vi "configure operation.vi"(7 "EthernetIP configuration":refnum<class "EthernetIP configuration.lvclass">, 8 "error in":errorcluster, 10 "line item in":T2, 11 "engine configuration in":refnum<class "engine configuration.lvclass">) -> (0 "error out":errorcluster, 1 "success":bool, 2 "line item out":T2, 5 "changed":bool)   [LabVIEW 2013, in "EthernetIP editor node.lvclass"]
uses:
  EthernetIP editor node.lvclass
  table line.ctl
  channel/EthernetIP Channel.lvclass
  <vilib>/NI/Module Execution Interface/Engine Configuration/engine configuration.lvclass
  configuration/EthernetIP configuration.lvclass
  <vilib>/NI/Tag Bus/tag/Data Type.ctl
  configuration/EthernetIP configuration.lvclass/EthernetIP configuration.ctl
  <vilib>/NI/Configuration Framework/serializable configuration/NISE_CEF_serializable configuration.lvclass/NISE_CEF_serializable configuration.ctl
  <vilib>/NI/Tag Bus/tag/tag descriptor.lvclass/tag descriptor.ctl
  channel/EthernetIP Channel.lvclass/EthernetIP Channel.ctl
  <vilib>/NI/Tag Bus Module Framework/channel/TBM channel.lvclass/TBM channel.ctl
  configuration/Read assemblies.vi
  <vilib>/NI/Configuration Framework/serializable configuration/Read UID.vi
  <vilib>/NI/Tag Bus Module Framework/channel/Read channel classification.vi
  <vilib>/NI/Tag Bus/tag/read tag name.vi
  <vilib>/NI/Tag Bus/tag/read data type.vi
  channel/Read byte index.vi
  channel/Read Instance ID.vi
  <vilib>/NI/Tag Bus/tag/write tag name.vi
  channel/Write Instance ID.vi
  <vilib>/NI/Tag Bus Module Framework/channel/Write channel classification.vi
  <vilib>/NI/Tag Bus/tag/write data type.vi
  channel/Write byte index.vi
  <vilib>/Utility/LVClass/Get LV Class Name.vi
  <vilib>/NI/Configuration Framework/error generator.vi
  <vilib>/NI/Tag Bus/tag/tag descriptor.lvclass
panel:
  out "Instance data type":T1=enum."Boolean"
  in  "refresh tags":bool
  in  "Tag":i32(listbox)
  in  "Instance":i32(listbox)
  out "problem":string
  in  "Element Index":i32
  in  "Channel Name":string
  in  "cancel":bool
  in  "ok":bool
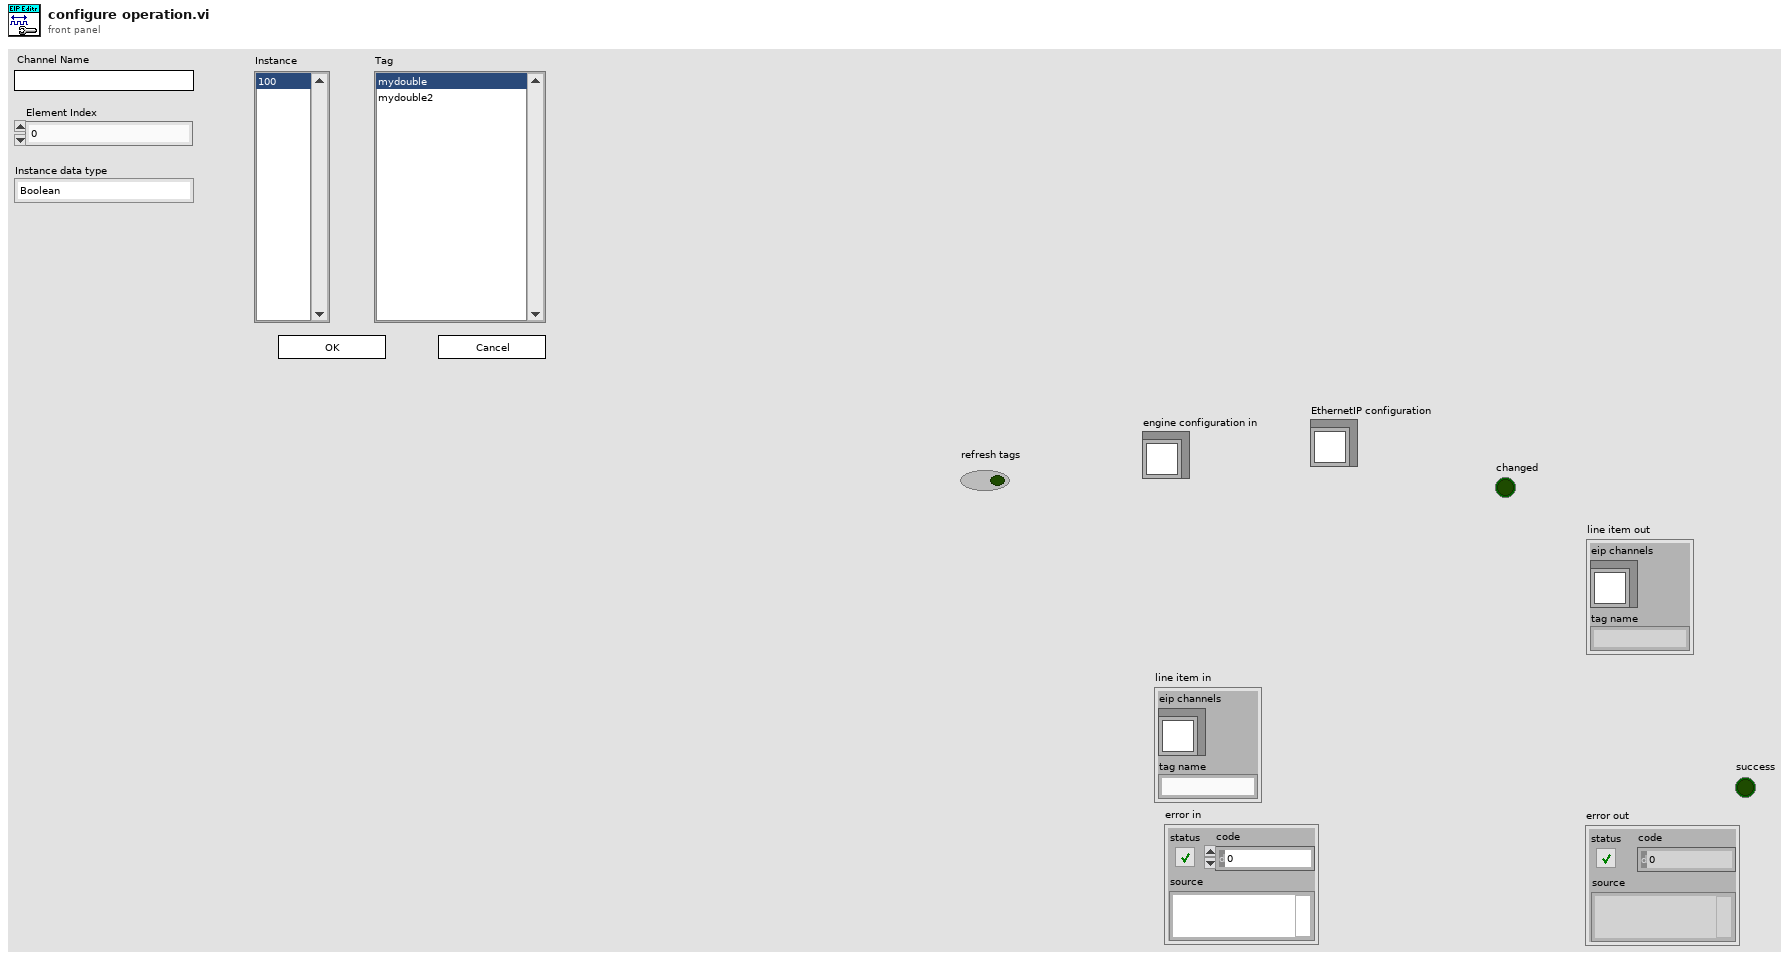
[diagram p1: front panel]
types:
  T1 = typedef "tag bus.lvlib/tag descriptor.lvclass/Data Type.ctl" = enum16{"Double", "Single", "I64", "I32", "I16", "I8", "U64", "U32", "U16", "U8", "Boolean", "String", "Array of Double", "Array of Single", "Array of I64", "Array of I32", "Array of I16", "Array of I8", "Array of U64", "Array of U32", "Array of U16", "Array of U8", "Array of Boolean", "Array of String"}
  T2 = typedef "EthernetIP editor node.lvclass/table line.ctl" = cluster{"eip channels":refnum<class "EthernetIP Channel.lvclass">, "tag name":string}
  T3 = enum32{"Invalid", "Standard", "Closed", "Hidden", "Minimized", "Maximized"}
  T4 = enum32{"Invalid", "Default", "Floating", "Floating/Auto-Hide", "Modal"}
  T5 = enum8{"Enabled", "Disabled", "Disabled and Grayed Out"}
  T6 = typedef "EthernetIP configuration.lvclass/assembly definition.ctl" = cluster{"name":string, "Instance ID":u32, "Type":T7, "Size (elements)":u32, "big endian?":bool, "data type":T1}
  T7 = typedef "EthernetIP configuration.lvclass/assembly type.ctl" = enum32{"Producing", "Consuming"}
  T8 = enum32{"invalid app kind", "Development System", "Run Time System", "Student Edition", "Embedded LabVIEW", "Evaluation", "Custom"}
  T9 = typedef "TBM channel.lvclass/channel classification.ctl" = enum16{"input data", "output data", "processing parameter", "processing result"}
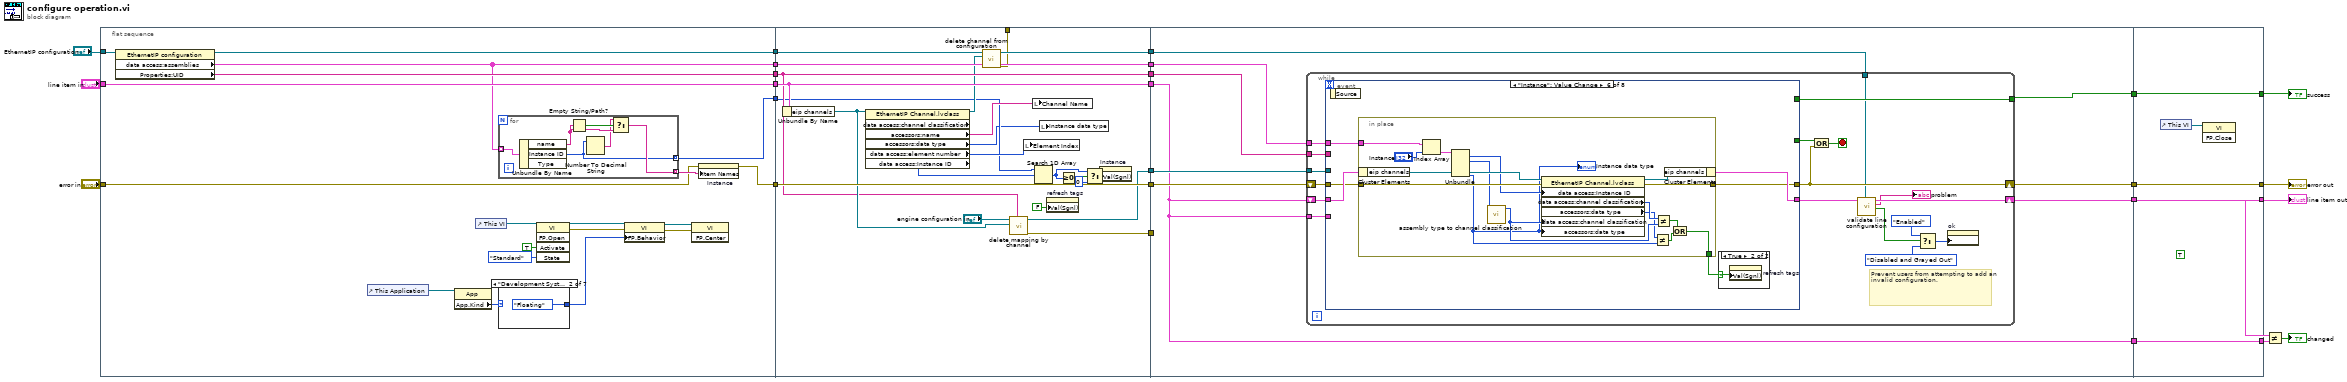
[diagram p0: block diagram]
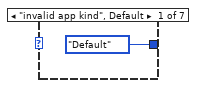
[diagram p2: hidden frame]
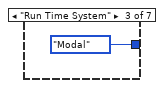
[diagram p3: hidden frame]
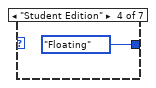
[diagram p4: hidden frame]
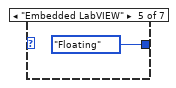
[diagram p5: hidden frame]
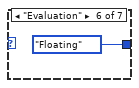
[diagram p6: hidden frame]
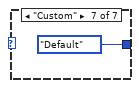
[diagram p7: hidden frame]
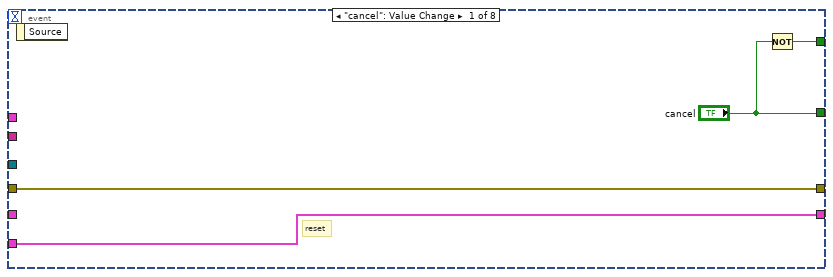
[diagram p8: hidden frame]
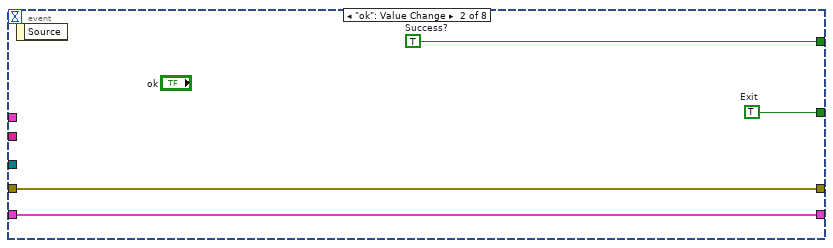
[diagram p9: hidden frame]
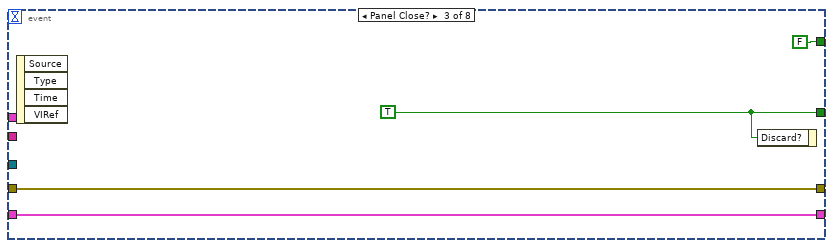
[diagram p10: hidden frame]
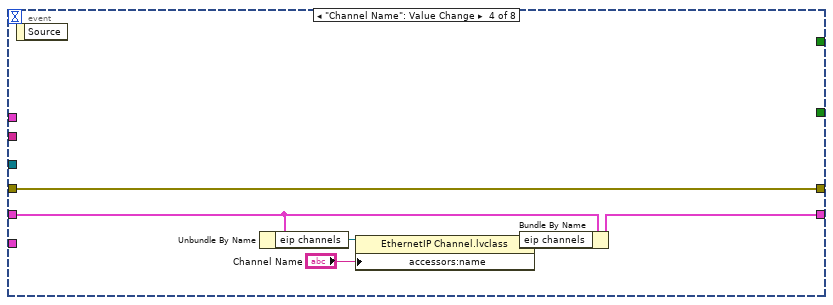
[diagram p11: hidden frame]
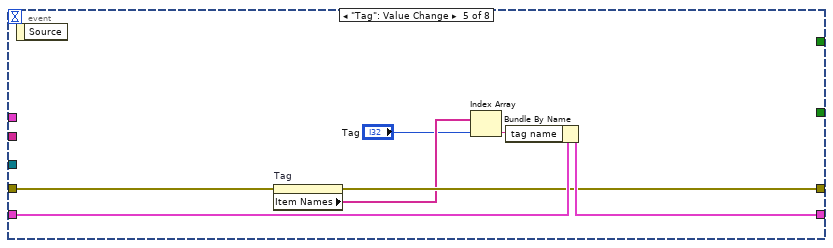
[diagram p12: hidden frame]
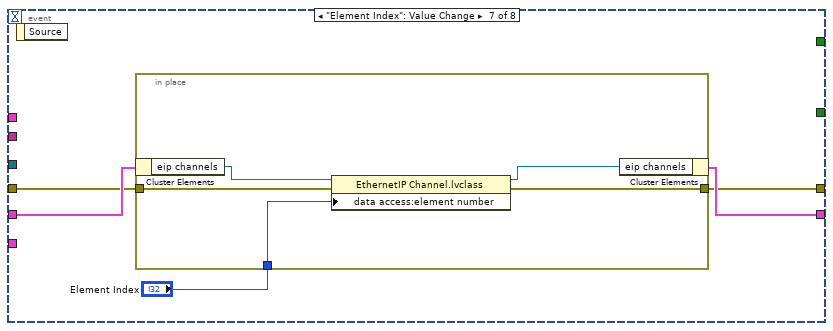
[diagram p14: hidden frame]
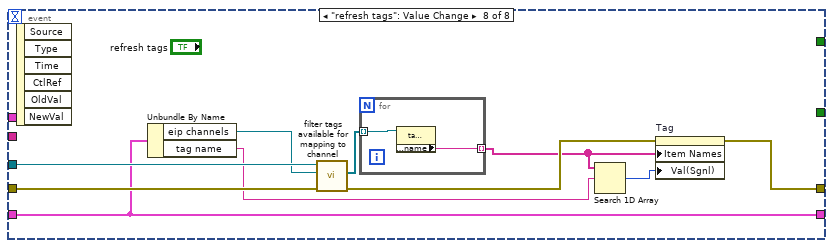
[diagram p15: hidden frame]
diagram:
  n1 = flat-sequence {
    tunnel: "line item in" -> [w44]
    tunnel: "error in" -> [w30]
    tunnel: [w29] -> w14
    tunnel: [w44] -> w12
    tunnel: "EthernetIP configuration" -> [w35]
    tunnel: [w34] -> w6
    tunnel: [w32] -> w4
    tunnel: [w33] -> w3
    tunnel: [w28] -> w1
    tunnel: w14 -> [w79]
    tunnel: [w79] -> w13
    tunnel: w12 -> [w77]
    tunnel: [w77] -> w11
    tunnel: [w75] -> w10
    tunnel: [w74] -> w9
    tunnel: [w68] -> w7
    tunnel: w6 -> [w71]
    tunnel: [w70] -> w5
    tunnel: w4 -> [w70]
    tunnel: w3 -> [w69]
    tunnel: [w69] -> w2
    tunnel: [w66] -> _
    tunnel: w1 -> [w65]
    tunnel: [w87] -> w18
    tunnel: [w86] -> w17
    tunnel: [w85] -> w16
    tunnel: [w80] -> w15
    tunnel: w13 -> [w88]
    tunnel: w11 -> [w80]
    tunnel: w10 -> [_]
    tunnel: w9 -> [w84]
    tunnel: w7 -> [w83]
    tunnel: w5 -> [w82]
    tunnel: w2 -> [w81]
    tunnel: [w177] -> w19
    tunnel: [w178] -> w22
    tunnel: [w179] -> w23
    tunnel: [w180] -> w24
    tunnel: w18 -> [w180]
    tunnel: w17 -> [w179]
    tunnel: w16 -> [w178]
    tunnel: w15 -> [w177]
    frame #0 {
      n2 = property class="EthernetIP configuration"(reference=w35) -> (reference out=w34:refnum<class "EthernetIP configuration.lvclass">, "data access:assemblies"=w32:T6[], "Properties:UID"=w33:string)  [unwired: 1 in, 1 out]
      n3 = control-ref of="This Application"() -> (w38:refnum<vi>)
      n4 = property class="App"(reference=w38) -> ("App.Kind"=w37:T8)  [unwired: 1 in, 2 out]
      n5 = control-ref of="This VI"() -> (w39:refnum<vi>)
      n6 = for {
        tunnel: w32 -> [w50] mode=indexing
        tunnel: [w46] -> w31 mode=indexing
        tunnel: [w45] -> w28 mode=indexing
        n7 = Unbundle By Name(w50) -> ("name"=w48:string, "Instance ID"=w45:u32)  [unwired: 1 out]
        n8 = Empty String/Path?(string/path=w48) -> (empty?=w49:bool)
        n9 = Number To Decimal String(number=w45) -> (decimal integer string=w47:string)  [unwired: 1 in]
        n10 = Select(t=w47, s=w49, f=w48) -> (s? t:f=w46:string)
      }
      n11 = case shown="\"Development System\"" w37 {
        tunnel: [T4."Default" ("Front Panel Window:Behavior") T4."Floating" ("Front Panel Window:Behavior") T4."Modal" ("Front Panel Window:Behavior") T4."Floating" ("Front Panel Window:Behavior") T4."Floating" ("Front Panel Window:Behavior") T4."Floating" ("Front Panel Window:Behavior") T4."Default" ("Front Panel Window:Behavior")] -> w36
        frame "invalid app kind", Default {
        }
        frame "Development System" {
        }
        frame "Run Time System" {
        }
        frame "Student Edition" {
        }
        frame "Embedded LabVIEW" {
        }
        frame "Evaluation" {
        }
        frame "Custom" {
        }
      }
      n12 = invoke class="VI" method="FP.Open"(reference=w39, "Activate"=TRUE ("Activate?"), "State"=T3."Standard") -> (reference out=w42:refnum<vi>, error out=w43:errorcluster)  [unwired: 2 in, 3 out]
      n13 = property class="VI"(reference=w42, error in=w43, "FP.Behavior"=w36) -> (reference out=w27:refnum<vi>, error out=w26:errorcluster)
      n14 = invoke class="VI" method="FP.Center"(reference=w27, error in=w26) -> ()  [unwired: 1 in, 3 out]
      n15 = property on="Instance" class="LstBox (strict)"(error in=w30, "Item Names"=w31) -> (error out=w29:errorcluster)  [unwired: 1 in, 1 out]
    }
    frame #1 {
      n16 = Unbundle By Name(w77) -> ("eip channels"=w73:refnum<class "EthernetIP Channel.lvclass">)
      n17 = property class="EthernetIP Channel.lvclass" props=["data access:channel classification", "accessors:name", "accessors:data type", "data access:element number", "data access:Instance ID"](reference=w73) -> (reference out=w67:refnum<class "EthernetIP Channel.lvclass">, "accessors:name"=w78:string, "accessors:data type"=w58:T1, "data access:element number"=w72:i32, "data access:Instance ID"=w60:u32)  [unwired: 1 in, 2 out]
      n18 = call "delete channel from configuration.vi"("TBM channel in"=w67, "EthernetIP configuration in"=w71) -> ("error out"=w66:errorcluster, "EthernetIP configuration out"=w68:refnum<class "EthernetIP configuration.lvclass">)  [unwired: 8 in]
      n19 = call <vilib>:"delete mapping by channel.vi"("owner ID"=w69, "channel"=w73, "engine configuration in"="engine configuration in") -> ("error out"=w75:errorcluster, "engine configuration out"=w74:refnum<class "engine configuration.lvclass">)  [unwired: 7 in]
      n20 = local write "Element Index"(w72) -> ()
      n21 = local write "Channel Name"(w78) -> ()
      n22 = Search 1D Array(1D array=w65, element=w60) -> (index of element=w62:i32)  [unwired: 1 in]
      n23 = local write "Instance data type"(w58) -> ()
      n24 = property on="refresh tags" class="Bool (strict)"("Val(Sgnl)"=FALSE ("Value (Signaling)")) -> ()  [unwired: 2 in, 2 out]
      n25 = Greater Or Equal To 0?(x=w62) -> (x >= 0?=w63:bool)
      n26 = Select(t=w62, s=w63, f=0) -> (s? t:f=w61:i32)
      n27 = property on="Instance" class="LstBox (strict)"("Val(Sgnl)"=w61) -> ()  [unwired: 2 in, 2 out]
    }
    frame #2 {
      n28 = while {
        shift-right: [w97] -> w86
        shift-left: w88 -> [w105]
        tunnel: [w104] -> w87
        shift-right: [w98] -> w85
        shift-left: w80 -> [w101]
        tunnel: w80 -> [w100]
        tunnel: w84 -> [w106]
        tunnel: w83 -> [w92]
        tunnel: w82 -> [w91]
        tunnel: w81 -> [w90]
        stop <- w102 stop-if-true
        # "Prevent users from attempting to add an invalid configuration."
        n29 = event shown="[5] \"Instance\": Value Change" {
          selector: _ -> [_ _ _ _ _ _ _ _]
          dyn-events: _ -> [_ _ _ _ _ _ _ _]
          timeout: _ -> [_ _ _ _ _ _ _ _]
          tunnel: w106 -> [_ _ _ _ _ _ _ w171]
          tunnel: w105 -> [w110 w114 w118 w124 w130 w135 w157 w173]
          tunnel: [w110 w114 w118 w124 w127 w134 w156 w172] -> w97
          tunnel: [w109 w111 FALSE _ _ _ _ _] -> w104
          tunnel: ["cancel" w112 w116 _ _ _ _ _] -> w103
          tunnel: w101 -> [_ w113 w115 w122 w131 w137 w159 w170]
          tunnel: [w107 w113 w115 w123 w129 w136 w158 w170] -> w99
          tunnel: w100 -> [w107 _ _ _ _ _ _ _]
          tunnel: w91 -> [_ _ _ _ _ w132 _ _]
          tunnel: w90 -> [_ _ _ _ _ _ _ _]
          event "cancel": Value Change {
            # "reset"
            n30 = event-data() -> ()  [unwired: 1 in, 1 out]
            n31 = Not(x="cancel") -> (.not. x?=w109:bool)
          }
          event "ok": Value Change {
            w111 = TRUE  # Success?
            w112 = TRUE  # Exit
            n32 = event-data() -> ()  [unwired: 1 in, 1 out]
          }
          event Panel Close? {
            w116 = TRUE ("cancel")
            n33 = event-data() -> ()  [unwired: 1 in, 4 out]
            n34 = event-data("Discard?"=w116) -> ()  [unwired: 1 in, 1 out]
          }
          event "Channel Name": Value Change {
            n35 = event-data() -> ()  [unwired: 1 in, 1 out]
            n36 = Unbundle By Name(w122) -> ("eip channels"=w121:refnum<class "EthernetIP Channel.lvclass">)
            n37 = property class="EthernetIP Channel.lvclass"(reference=w121, "accessors:name"="Channel Name") -> (reference out=w120:refnum<class "EthernetIP Channel.lvclass">)  [unwired: 1 in, 1 out]
            n38 = Bundle By Name(cluster=w122, "eip channels"=w120) -> (w123:T2)
          }
          event "Tag": Value Change {
            n39 = event-data() -> ()  [unwired: 1 in, 1 out]
            n40 = property on="Tag" class="LstBox (strict)"(error in=w130) -> (error out=w127:errorcluster, "Item Names"=w126:string[])  [unwired: 1 in, 1 out]
            n41 = Index Array(array=w126, index="Tag") -> (element=w128:string)
            n42 = Bundle By Name(cluster=w131, "tag name"=w128) -> (w129:T2)
          }
          event "Instance": Value Change {
            n43 = event-data() -> ()  [unwired: 1 in, 1 out]
            n44 = in-place {
              in-place-border: w135 -> [w154]
              in-place-border: [w153] -> w134
              in-place-border: [w140] -> w133
              in-place-border: w132 -> [w147]
              n45 = in-place-cluster #1(w137) -> ("eip channels"=w152:refnum<class "EthernetIP Channel.lvclass">)
              n46 = Index Array(array=w147, index="Instance") -> (element=w146:T6)
              n47 = Unbundle(w146) -> ("Instance ID"=w145:u32, "Type"=w144:T7, "data type"=w139:T1)  [unwired: 3 out]
              "Instance data type" <- w139
              n48 = call "assembly type to channel classification.vi"("Type"=w144) -> ("channel classification"=w149:T9)  [unwired: 10 in]
              n49 = property class="EthernetIP Channel.lvclass"(reference=w152, error in=w154, "data access:Instance ID"=w145, "data access:channel classification"=w149, "accessors:data type"=w139) -> (reference out=w151:refnum<class "EthernetIP Channel.lvclass">, error out=w153:errorcluster, "data access:channel classification"=w150:T9, "accessors:data type"=w143:T1)
              n50 = Not Equal?(x=w143, y=w139) -> (x != y?=w142:bool)
              n51 = Not Equal?(x=w150, y=w149) -> (x != y?=w141:bool)
              n52 = in-place-cluster #1("eip channels"=w151) -> (w136:T2)
              n53 = Or(x=w141, y=w142) -> (x .or. y?=w140:bool)
            }
            n54 = case shown="True" w133 {
              selector: w133 -> [_ w138]
              frame False {
              }
              frame True {
                n55 = property on="refresh tags" class="Bool (strict)"("Val(Sgnl)"=w138) -> ()  [unwired: 2 in, 2 out]
              }
            }
          }
          event "Element Index": Value Change {
            n56 = event-data() -> ()  [unwired: 1 in, 1 out]
            n57 = in-place {
              in-place-border: w157 -> [w164]
              in-place-border: [w163] -> w156
              in-place-border: "Element Index" -> [w160]
              n58 = in-place-cluster #2(w159) -> ("eip channels"=w162:refnum<class "EthernetIP Channel.lvclass">)
              n59 = property class="EthernetIP Channel.lvclass"(reference=w162, error in=w164, "data access:element number"=w160) -> (reference out=w161:refnum<class "EthernetIP Channel.lvclass">, error out=w163:errorcluster)
              n60 = in-place-cluster #2("eip channels"=w161) -> (w158:T2)
            }
          }
          event "refresh tags": Value Change {
            n61 = event-data() -> ()  [unwired: 1 in, 6 out]
            n62 = Unbundle By Name(w170) -> ("eip channels"=w169:refnum<class "EthernetIP Channel.lvclass">, "tag name"=w166:string)
            n63 = call <vilib>:"filter tags available for mapping to channel.vi"("channel to map to"=w169, "engine configuration in"=w171) -> ("filtered tags"=w168:refnum<class "tag descriptor.lvclass">[])  [unwired: 8 in, 1 out]
            n64 = for {
              tunnel: w168 -> [w175] mode=indexing
              tunnel: [w174] -> w167 mode=indexing
              n65 = property class="tag descriptor"(reference=w175) -> ("accessors:name"=w174:string)  [unwired: 1 in, 2 out]
            }
            n66 = Search 1D Array(1D array=w167, element=w166) -> (index of element=w165:i32)  [unwired: 1 in]
            n67 = property on="Tag" class="LstBox (strict)"(error in=w173, "Item Names"=w167, "Val(Sgnl)"=w165) -> (error out=w172:errorcluster)  [unwired: 1 in, 1 out]
          }
        }
        n68 = Compound Arithmetic op=OR(w103, w97) -> (w102:bool)
        n69 = call "validate line configuration.vi"("EthernetIP configuration"=w92, "line in"=w99) -> ("valid?"=w96:bool, "problem"=→"problem":string, "line out"=w98:T2)  [unwired: 7 in]
        n70 = Select(t=T5."Enabled" ("Disabled"), s=w96, f=T5."Disabled and Grayed Out") -> (s? t:f=w93:T5)
        n71 = property on="ok" class="Bool"("DisabledEnum"=w93) -> ()  [unwired: 2 in, 2 out]
      }
    }
    frame #3 {
      (unwired) TRUE ("Visible")
      n72 = control-ref of="This VI"() -> (w176:refnum<vi>)
      n73 = invoke class="VI" method="FP.Close"(reference=w176) -> ()  [unwired: 2 in, 3 out]
    }
  }
  n74 = Not Equal?(x=w22, y=w19) -> (x != y?=→"changed":bool)
  "error out" <- w23
  "success" <- w24
  "line item out" <- w22
